vi "CALC_MARK_DELT_ON_OFF.vi"(0 "VISA IN":refnum<visa-resource-name>, 1 "Marker number":i32, 2 "Marker is Delta(ON) or Absolute(OFF)":bool, 5 "error in":errorcluster, 7 "Channel":i32) -> (14 "VISA Out":refnum<visa-resource-name>, 19 "error out":errorcluster)   [LabVIEW 2018, in "PNA-X.lvlib"]
doc: "CALCulate<cnum>:MARKer<mkr>:DELTa <ON|OFF> \n1529\n\n(Read-Write) Specifies whether marker is relative to the Reference marker or absolute. \nNote: The reference marker must already be turned ON with CALC:MARK:REF:STATE. \nSee Critical Note \nParameters \n<cnum> Channel number of the measurement. There must be a selected measurement \non that channel. If unspecified, <cnum> is set to 1. \n<mkr> Any existing marker number from 1 to 10; if unspecified, value is set to 1. \n<ON|OFF> ON (or 1) - Specified marker is a Delta marker \nOFF (or 0) - Specified marker is an ABSOLUTE marker \nExamples CALC:MARK:DELT ON \ncalculate2:marker8:delta off \nQuery Syntax CALCulate<cnum>:MARKer<mkr>:DELTa? \nReturn Type Boolean (1 = ON, 0 = OFF) \nDefault OFF"
uses:
  PNA-X.lvlib
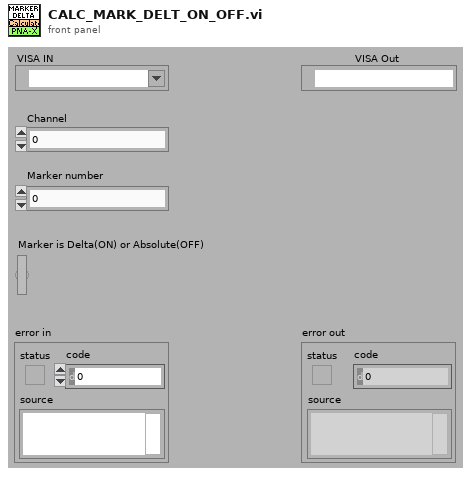
[diagram p1: front panel]
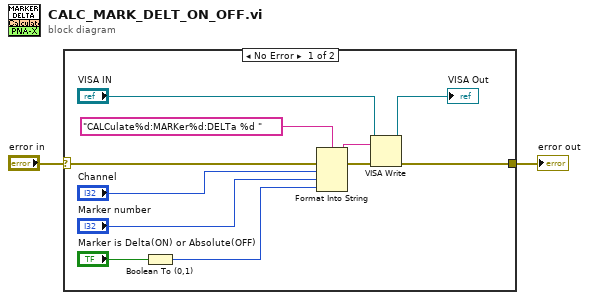
[diagram p0: block diagram]
diagram:
  n1 = case shown="No Error" "error in" {
    selector: "error in" -> [w13 w14]
    tunnel: [w8 w14] -> w1
    frame No Error {
      n2 = Boolean To (0,1)(Boolean="Marker is Delta(ON) or Absolute(OFF)") -> (0, 1=w3:i16)
      n3 = Format Into String(format string="CALCulate%d:MARKer%d:DELTa %d " ("Cmdline"), error in=w13, "Channel", "Marker number", w3) -> (resulting string=w11:string, error out=w12:errorcluster)  [unwired: 1 in]
      n4 = VISA Write(VISA resource name="VISA IN", write buffer=w11, error in (no error)=w12) -> (VISA resource name out=→"VISA Out":refnum<visa-resource-name>, error out=w8:errorcluster)  [unwired: 1 out]
    }
    frame Error {
    }
  }
  "error out" <- w1
